vi "output.vi"(8 "error in":errorcluster, 10 "data table in":T1, 11 "Shared Memory runtime in":refnum<class "Shared Memory runtime.lvclass">) -> (0 "error out":errorcluster, 2 "data table out":T1, 3 "Shared Memory runtime out":refnum<class "Shared Memory runtime.lvclass">)   [LabVIEW 2014, in "Shared Memory runtime.lvclass"]
doc: "Provides an interface for writing data to a module at runtime. While this interface performs no operations, a child should provide an override which may write to any open sessions, references, or interfaces."
uses:
  Shared Memory runtime.lvclass
  <vilib>/NI/Tag Bus/table/data table.ctl
  <vilib>/NI/Tag Bus Module Framework/channel/channel classification.ctl
  Shared Memory runtime.lvclass/Shared Memory runtime.ctl
  <vilib>/NI/NI Linux RT IPC/Shared Memory/Pointer Operations/Read 1D Array DBL.vi
  <vilib>/NI/Tag Bus/table/write multiple elements.vi
  <vilib>/NI/Tag Bus/table/data polymorphs/write many/write Doubles.vi
  <vilib>/NI/NI Linux RT IPC/Shared Memory/Pointer Operations/Read 1D Array SGL.vi
  <vilib>/NI/Tag Bus/table/data polymorphs/write many/write Singles.vi
  <vilib>/NI/NI Linux RT IPC/Shared Memory/Pointer Operations/Read 1D Array I64.vi
  <vilib>/NI/Tag Bus/table/data polymorphs/write many/write I64s.vi
  <vilib>/NI/NI Linux RT IPC/Shared Memory/Pointer Operations/Read 1D Array I32.vi
  <vilib>/NI/Tag Bus/table/data polymorphs/write many/write I32s.vi
  <vilib>/NI/NI Linux RT IPC/Shared Memory/Pointer Operations/Read 1D Array I16.vi
  <vilib>/NI/Tag Bus/table/data polymorphs/write many/write I16s.vi
  <vilib>/NI/NI Linux RT IPC/Shared Memory/Pointer Operations/Read 1D Array I8.vi
  <vilib>/NI/Tag Bus/table/data polymorphs/write many/write I8s.vi
  <vilib>/NI/NI Linux RT IPC/Shared Memory/Pointer Operations/Read 1D Array U64.vi
  <vilib>/NI/Tag Bus/table/data polymorphs/write many/write U64s.vi
  <vilib>/NI/NI Linux RT IPC/Shared Memory/Pointer Operations/Read 1D Array U32.vi
  <vilib>/NI/Tag Bus/table/data polymorphs/write many/write U32s.vi
  <vilib>/NI/NI Linux RT IPC/Shared Memory/Pointer Operations/Read 1D Array U16.vi
  <vilib>/NI/Tag Bus/table/data polymorphs/write many/write U16s.vi
  <vilib>/NI/NI Linux RT IPC/Shared Memory/Pointer Operations/Read 1D Array U8.vi
  <vilib>/NI/Tag Bus/table/data polymorphs/write many/write U8s.vi
  <vilib>/NI/NI Linux RT IPC/Shared Memory/Pointer Operations/Read 1D Array Boolean.vi
  <vilib>/NI/Tag Bus/table/data polymorphs/write many/write Booleans.vi
  <vilib>/NI/Tag Bus/table/write sequential data elements.vi
  <vilib>/NI/Tag Bus/table/data polymorphs/write sequential/write sequential Doubles.vi
  <vilib>/NI/Tag Bus/table/data polymorphs/write sequential/write sequential Singles.vi
  <vilib>/NI/Tag Bus/table/data polymorphs/write sequential/write sequential I64s.vi
  <vilib>/NI/Tag Bus/table/data polymorphs/write sequential/write sequential I32s.vi
  <vilib>/NI/Tag Bus/table/data polymorphs/write sequential/write sequential I16s.vi
  <vilib>/NI/Tag Bus/table/data polymorphs/write sequential/write sequential I8s.vi
  <vilib>/NI/Tag Bus/table/data polymorphs/write sequential/write sequential U64s.vi
  <vilib>/NI/Tag Bus/table/data polymorphs/write sequential/write sequential U32s.vi
  <vilib>/NI/Tag Bus/table/data polymorphs/write sequential/write sequential U16s.vi
  <vilib>/NI/Tag Bus/table/data polymorphs/write sequential/write sequential U8s.vi
  <vilib>/NI/Tag Bus/table/data polymorphs/write sequential/write sequential Booleans.vi
  read channels of classification.vi
  Read input data.vi
  Read processing parameters.vi
  Read processing results.vi
  Read output data.vi
  <vilib>/NI/NI Linux RT IPC/Shared Memory/Classes/Shared Memory/Shared Memory.lvclass
  <vilib>/NI/Tag Bus Module Framework/channel/TBM channel.lvclass
  <vilib>/NI/Tag Bus/table/data table.lvlib
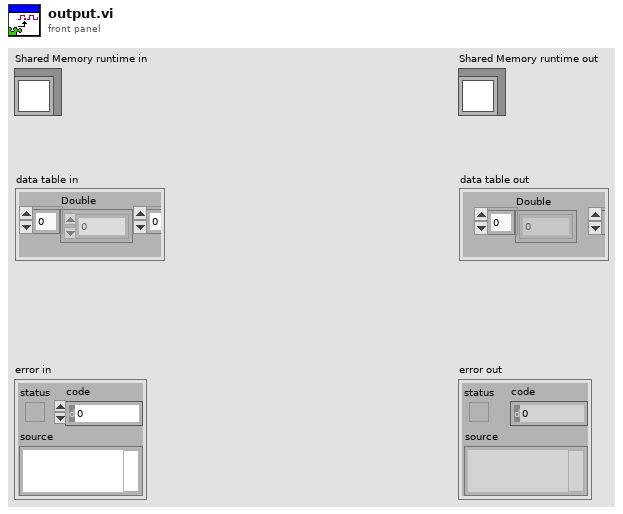
[diagram p1: front panel]
types:
  T1 = typedef "tag bus.lvlib/data table.lvlib/data table.ctl" = cluster{"Double":dbl[], "Single":sgl[], "I64":i64[], "I32":i32[], "I16":i16[], "I8":i8[], "U64":u64[], "U32":u32[], "U16":u16[], "U8":u8[], "Boolean":bool[], "String":string[], "Array of Double":cluster{"DBL Array":dbl[]}[], "Array of Single":cluster{"SGL Array":sgl[]}[], "Array of I64":cluster{"I64 Array":i64[]}[], "Array of I32":cluster{"I32 Array":i32[]}[], "Array of I16":cluster{"I16 Array":i16[]}[], "Array of I8":cluster{"I8 Array":i8[]}[], "Array of U64":cluster{"U64 Array":u64[]}[], "Array of U32":cluster{"U32 Array":u32[]}[], "Array of U16":cluster{"U16 Array":u16[]}[], "Array of U8":cluster{"U8 Array":u8[]}[], "Array of Boolean":cluster{"Boolean Array":bool[]}[], "Array of String":cluster{"String Array":string[]}[]}
  T2 = typedef "TBM channel.lvclass/channel classification.ctl" = enum16{"input data", "output data", "processing parameter", "processing result"}
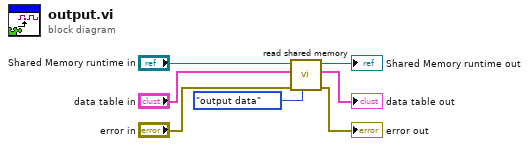
[diagram p0: block diagram]
diagram:
  n1 = call "read shared memory.vi"("channel classification"=channel_classification."output data", "error in"="error in", "data table"="data table in", "Shared Memory runtime"="Shared Memory runtime in") -> ("error out"=→"error out":errorcluster, "data table out"=→"data table out":T1, "Shared Memory runtime out"=→"Shared Memory runtime out":refnum<class "Shared Memory runtime.lvclass">)  [unwired: 5 in]
